vi "OpenConnection.vi"(6 "timeout hand shake [ms]":i32=5000, 7 "timeout opening [ms]":i32=5000, 8 "error in (no error)":errorcluster, 9 "WS Server Port":string="25010", 10 "WS Server IP":string="ws://127.0.0.1", 11 "Communicator in":refnum<class "Communicator.lvclass">) -> (0 "error out":errorcluster, 2 "Return Headers":variant, 3 "Communicator out":refnum<class "Communicator.lvclass">)   [LabVIEW 2020, in "horiba.lvlib" / "Communicator.lvclass"]
doc: "Opens a connection to the ICL via werbsocket."
uses:
  Communicator.lvclass
  Communicator.lvclass/Communicator.ctl
  <vilib>/MediaMongrels Ltd/WebSockets/WebSockets/WebSocket/WebSocket.lvclass/WebSocket.ctl
  <vilib>/MediaMongrels Ltd/WebSockets/WebSockets/WebSocket Client/WebSocket Client.lvclass
  C:/Program Files (x86)/National Instruments/LabVIEW 2024/vi.lib/MediaMongrels Ltd/WebSockets/WebSockets/WebSocket/WebSocket.lvclass
  <vilib>/MediaMongrels Ltd/WebSockets/WebSockets/WebSocket/WebSocket.lvclass
panel:
  # "Connector Pane"
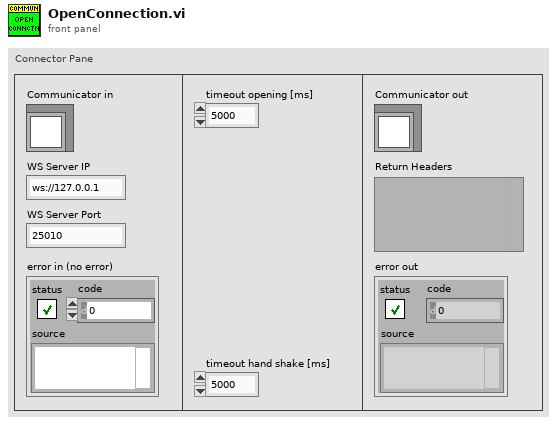
[diagram p1: front panel]
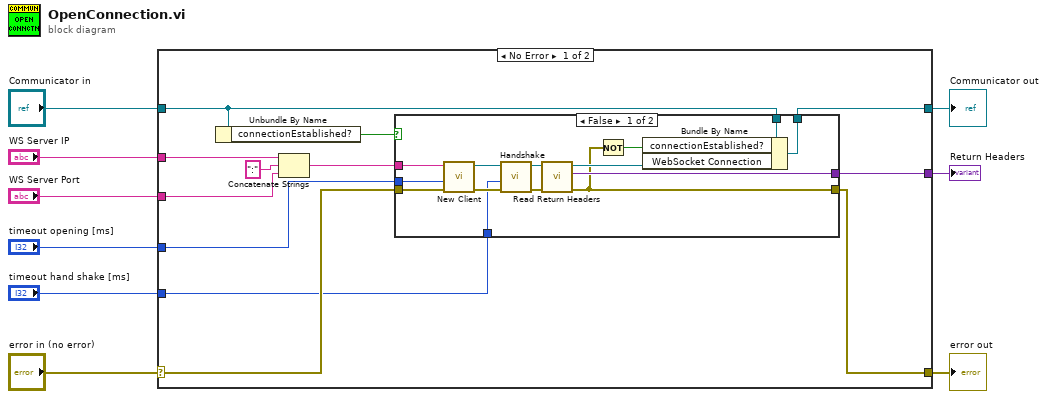
[diagram p0: block diagram]
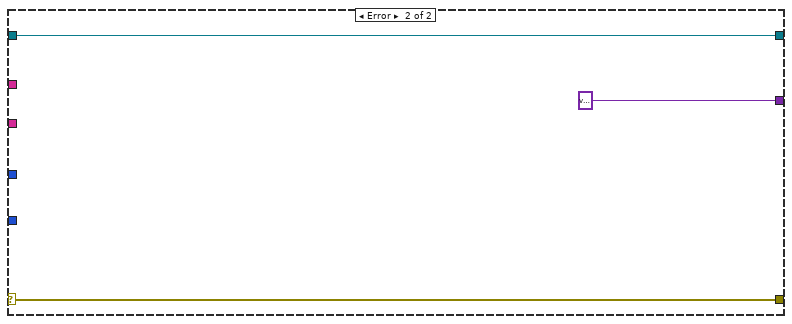
[diagram p3: hidden frame]
diagram:
  n1 = case shown="No Error" "error in (no error)" {
    selector: "error in (no error)" -> [w21 w40]
    tunnel: [w20 w40] -> w8
    tunnel: [w19 w39] -> w6
    tunnel: "Communicator in" -> [w11 w39]
    tunnel: "WS Server IP" -> [w17 _]
    tunnel: "WS Server Port" -> [w16 _]
    tunnel: [w14 variant ("Return Headers")] -> w3
    tunnel: "timeout opening [ms]" -> [w13 _]
    tunnel: "timeout hand shake [ms]" -> [w12 _]
    frame No Error {
      n2 = Unbundle By Name(w11) -> ("connectionEstablished?"=w10:bool)
      n3 = Concatenate Strings(w17, ":" ("string"), w16) -> (w15:string)
      n4 = case shown="False" w10 {
        tunnel: w21 -> [w33 w36]
        tunnel: [w22 w36] -> w20
        tunnel: [w32 w37] -> w19
        tunnel: w15 -> [w28 _]
        tunnel: [w27 _] -> w14
        tunnel: w13 -> [w26 _]
        tunnel: w12 -> [w25 _]
        tunnel: w11 -> [w24 w37]
        frame False {
          n5 = call <vilib>:"New Client.vi"("error in (no error)"=w33, "timeout ms (5000)"=w26, "WebSocket URL"=w28) -> ("error out"=w30:errorcluster, "WebSocket Client out"=w35:refnum<class "WebSocket Client.lvclass">)  [unwired: 7 in]
          n6 = call-dynamic "Handshake.vi"("error in (no error)"=w30, "timeout ms (5000)"=w25, "WebSocket Client in"=w35) -> ("error out"=w29:errorcluster, "WebSocket Client out"=w34:refnum<class "WebSocket Client.lvclass">)  [unwired: 7 in]
          n7 = call <vilib>:"Read Return Headers.vi"("error in (no error)"=w29, "WebSocket in"=w34) -> ("error out"=w22:errorcluster, "Return Headers"=w27:variant, "WebSocket out"=w31:refnum<class "WebSocket Client.lvclass">)  [unwired: 7 in]
          n8 = Not(x=w22) -> (.not. x?=w23:bool)
          n9 = Bundle By Name(cluster=w24, "connectionEstablished?"=w23, "WebSocket Connection"=w31) -> (w32:refnum<class "Communicator.lvclass">)
        }
        frame True {
        }
      }
    }
    frame Error {
    }
  }
  "error out" <- w8
  "Communicator out" <- w6
  "Return Headers" <- w3
